vi "path.get.vi"(8 "error in (no error)":errorcluster, 11 "source in":refnum<class "source.lvclass">) -> (0 "error out":errorcluster, 2 "path":string, 3 "source out":refnum<class "source.lvclass">)   [LabVIEW 2020, in "datasources.lvlib" / "source.lvclass"]
uses:
  source.lvclass
  source.lvclass/source.ctl
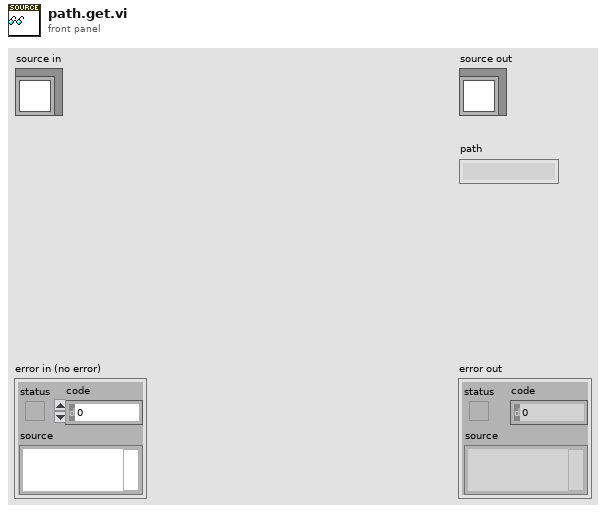
[diagram p1: front panel]
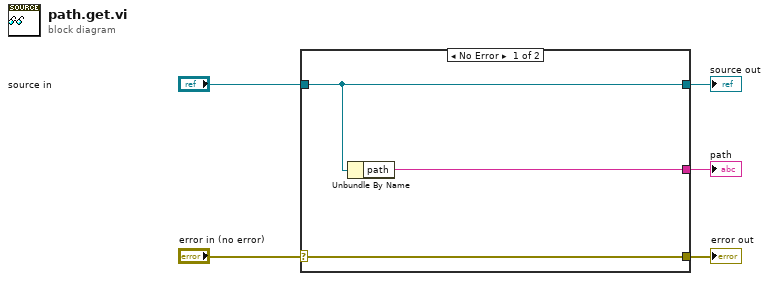
[diagram p0: block diagram]
diagram:
  n1 = case shown="No Error" "error in (no error)" {
    selector: "error in (no error)" -> [w8 w9]
    tunnel: [w8 w9] -> w4
    tunnel: [w7 w10] -> w2
    tunnel: "source in" -> [w7 w10]
    tunnel: [w6 _] -> w1
    frame No Error {
      n2 = Unbundle By Name(w7) -> ("path"=w6:string)
    }
    frame Error {
    }
  }
  "error out" <- w4
  "source out" <- w2
  "path" <- w1
